vi "System Explorer - Add content to System Explorer library.vi"(8 "error in (no error)":errorcluster, 11 "CD Wizard - Internal Data IN":T1) -> (0 "error out":errorcluster)   [LabVIEW 2015]
doc: "Add all virtual folders and VIs to the System Explorer library."
uses:
  TypDef/CD Wizard - Internal data.ctl
  TypDef/CD Wizard - Execution Mode.ctl
  TypDef/CD Wizard - Extra Page Name and GUID.ctl
  Constants/Constants TypDef/CD System Explorer lvlib.ctl
  TypDef/Add Item - Type.ctl
  Constants/CD System Explorer lvlib.vi
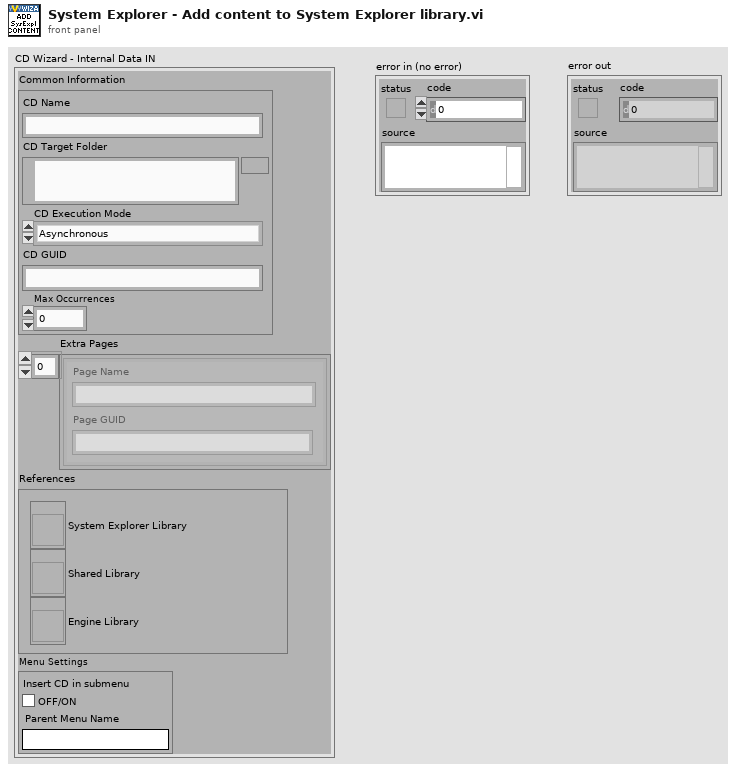
[diagram p1: front panel]
types:
  T1 = typedef "CD Wizard - Internal data.ctl" = cluster{"Common Information":cluster{"CD Name":string, "CD Target Folder":path, "CD Execution Mode":T2, "CD GUID":string, "Max Occurrences":u32}, "Extra Pages":T3[], "References":cluster{"System Explorer Library":refnum<vi>, "Shared Library":refnum<vi>, "Engine Library":refnum<vi>}, "Menu Settings":cluster{"Insert CD in submenu":bool, "Parent Menu Name":string}}
  T2 = typedef "CD Wizard - Execution Mode.ctl" = enum16{"Asynchronous", "Inline HW Interface", "Inline Model Interface", "Inline Timing and Sync", "Asynchronous Timing and Sync"}
  T3 = typedef "CD Wizard - Extra Page Name and GUID.ctl" = cluster{"Page Name":string, "Page GUID":string}
  T4 = typedef "CD System Explorer lvlib.ctl" = enum16{"LibraryFileName", "LibraryFolderName", "System Explorer.FolderName", "System Explorer.Dynamically Called.FolderName", "System Explorer.Dynamically Called.Extra Pages.FolderName", "System Explorer.Dynamically Called.Extra Pages.TemplatePathAndName", "System Explorer.Dynamically Called.Main Page.VIName", "System Explorer.Dynamically Called.Main Page.TemplatePathAndName", "System Explorer.Dynamically Called.Initialization VI.VIName", "System Explorer.Dynamically Called.Initialization VI.TemplatePathAndName", "System Explorer.SubVI.FolderName", "System Explorer.Types.FolderName", "System Explorer.ActionVIOnCompile.VIName", "System Explorer.ExportConfigRTM.VIName"}
  T5 = typedef "Add Item - Type.ctl" = string
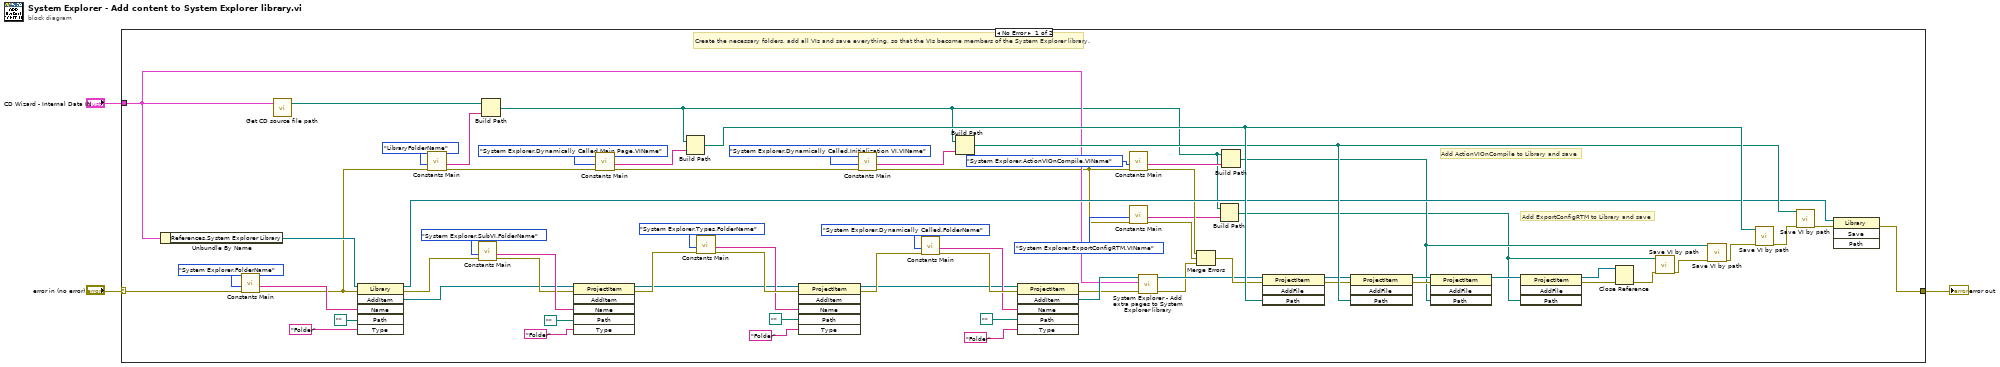
[diagram p0: block diagram]
diagram:
  n1 = case shown="No Error" "error in (no error)" {
    selector: "error in (no error)" -> [w72 w73]
    tunnel: "CD Wizard - Internal Data IN" -> [w27 _]
    tunnel: [w71 w73] -> w1
    frame No Error {
      # "Add ExportConfigRTM to Library and save"
      # "Add ActionVIOnCompile to Library and save"
      # "Create the necessary folders, add all VIs and save everything, so that the VIs become members of the System Explorer library."
      n2 = Unbundle By Name(w27) -> ("References.System Explorer Library"=w33:refnum<vi>)
      n3 = call-poly "Constants Main.vi"("error in (no error)"=w72, "Action"=CD_System_Explorer_lvlib."System Explorer.FolderName") -> ("error out"=w23:errorcluster, "Output"=w67:string)  [unwired: 8 in]
      n4 = call "Get CD source file path.vi"("CD Wizard - Internal Data"=w27) -> ("CD Source file path"=w32:path)  [unwired: 2 in]
      n5 = invoke class="Library" method="AddItem"(reference=w33, error in=w23, "Name"=w67, "Path"=path "", "Type"=T5 "Folder" ("Add Item - Type")) -> (reference out=w35:refnum<vi>, error out=w47:errorcluster, "AddItem"=w34:refnum<vi>)  [unwired: 1 in, 3 out]
      n6 = call-poly "Constants Main.vi"("error in (no error)"=w23, "Action"=CD_System_Explorer_lvlib."LibraryFolderName") -> ("error out"=w24:errorcluster, "Output"=w22:string)  [unwired: 8 in]
      n7 = call-poly "Constants Main.vi"("error in (no error)"=w47, "Action"=CD_System_Explorer_lvlib."System Explorer.SubVI.FolderName") -> ("error out"=w55:errorcluster, "Output"=w57:string)  [unwired: 8 in]
      n8 = Build Path(base path=w32, name or relative path=w22) -> (appended path=w5:path)
      n9 = invoke class="ProjectItem" method="AddItem"(reference=w34, error in=w55, "Name"=w57, "Path"=path "", "Type"=T5 "Folder" ("Add Item - Type")) -> (reference out=w39:refnum<vi>, error out=w46:errorcluster)  [unwired: 1 in, 4 out]
      n10 = call-poly "Constants Main.vi"("error in (no error)"=w24, "Action"=CD_System_Explorer_lvlib."System Explorer.Dynamically Called.Main Page.VIName") -> ("error out"=w26:errorcluster, "Output"=w65:string)  [unwired: 8 in]
      n11 = Build Path(base path=w5, name or relative path=w65) -> (appended path=w60:path)
      n12 = call-poly "Constants Main.vi"("error in (no error)"=w46, "Action"=CD_System_Explorer_lvlib."System Explorer.Types.FolderName") -> ("error out"=w52:errorcluster, "Output"=w50:string)  [unwired: 8 in]
      n13 = invoke class="ProjectItem" method="AddItem"(reference=w39, error in=w52, "Name"=w50, "Path"=path "", "Type"=T5 "Folder" ("Add Item - Type")) -> (reference out=w37:refnum<vi>, error out=w38:errorcluster)  [unwired: 1 in, 4 out]
      n14 = call-poly "Constants Main.vi"("error in (no error)"=w26, "Action"=CD_System_Explorer_lvlib."System Explorer.Dynamically Called.Initialization VI.VIName") -> ("error out"=w9:errorcluster, "Output"=w64:string)  [unwired: 8 in]
      n15 = call-poly "Constants Main.vi"("error in (no error)"=w38, "Action"=CD_System_Explorer_lvlib."System Explorer.Dynamically Called.FolderName") -> ("error out"=w44:errorcluster, "Output"=w42:string)  [unwired: 8 in]
      n16 = Build Path(base path=w5, name or relative path=w64) -> (appended path=w59:path)
      n17 = invoke class="ProjectItem" method="AddItem"(reference=w37, error in=w44, "Name"=w42, "Path"=path "", "Type"=T5 "Folder" ("Add Item - Type")) -> (error out=w29:errorcluster, "AddItem"=w31:refnum<vi>)  [unwired: 1 in, 4 out]
      n18 = call-poly "Constants Main.vi"("error in (no error)"=w9, "Action"=CD_System_Explorer_lvlib."System Explorer.ActionVIOnCompile.VIName") -> ("error out"=w8:errorcluster, "Output"=w16:string)  [unwired: 8 in]
      n19 = call-poly "Constants Main.vi"("error in (no error)"=w9, "Action"=CD_System_Explorer_lvlib."System Explorer.ExportConfigRTM.VIName") -> ("error out"=w7:errorcluster, "Output"=w6:string)  [unwired: 8 in]
      n20 = call "System Explorer - Add extra pages to System Explorer library.vi"("error in (no error)"=w29, "CD Wizard - Internal Data"=w27, "ProjectItem IN"=w31) -> ("error out"=w28:errorcluster, "ProjectItem OUT"=w30:refnum<vi>)  [unwired: 7 in]
      n21 = Merge Errors(w8, w7, w28) -> (w36:errorcluster)
      n22 = Build Path(base path=w5, name or relative path=w6) -> (appended path=w4:path)
      n23 = Build Path(base path=w5, name or relative path=w16) -> (appended path=w18:path)
      n24 = invoke class="ProjectItem" method="AddFile"(reference=w30, error in=w36, "Path"=w60) -> (reference out=w40:refnum<vi>, error out=w41:errorcluster)  [unwired: 1 in, 2 out]
      n25 = invoke class="ProjectItem" method="AddFile"(reference=w40, error in=w41, "Path"=w59) -> (reference out=w21:refnum<vi>, error out=w20:errorcluster)  [unwired: 1 in, 2 out]
      n26 = invoke class="ProjectItem" method="AddFile"(reference=w21, error in=w20, "Path"=w18) -> (reference out=w15:refnum<vi>)  [unwired: 1 in, 3 out]
      n27 = invoke class="ProjectItem" method="AddFile"(reference=w15, "Path"=w4) -> (reference out=w14:refnum<vi>, error out=w13:errorcluster)  [unwired: 2 in, 2 out]
      n28 = Close Reference(reference=w14, error in (no error)=w13) -> (error out=w11:errorcluster)
      n29 = call "Save VI by path.vi"("error in (no error)"=w11, "VI path"=w4) -> ("error out"=w12:errorcluster)  [unwired: 9 in]
      n30 = call "Save VI by path.vi"("error in (no error)"=w12, "VI path"=w18) -> ("error out"=w19:errorcluster)  [unwired: 9 in]
      n31 = call "Save VI by path.vi"("error in (no error)"=w19, "VI path"=w60) -> ("error out"=w62:errorcluster)  [unwired: 9 in]
      n32 = call "Save VI by path.vi"("error in (no error)"=w62, "VI path"=w59) -> ("error out"=w61:errorcluster)  [unwired: 9 in]
      n33 = invoke class="Library" method="Save"(reference=w35, error in=w61) -> (error out=w71:errorcluster)  [unwired: 2 in, 3 out]
    }
    frame Error {
      # "Output default values."
    }
  }
  "error out" <- w1
